vi "TelemetryServer_ChannelList.vi"(2 "error out":errorcluster, 3 "serverName":string) -> (0 "error in (no error)":errorcluster, 1 "Channel List":string[](array[string]))   [LabVIEW 2009]
uses:
  lib/lvrtc.dll
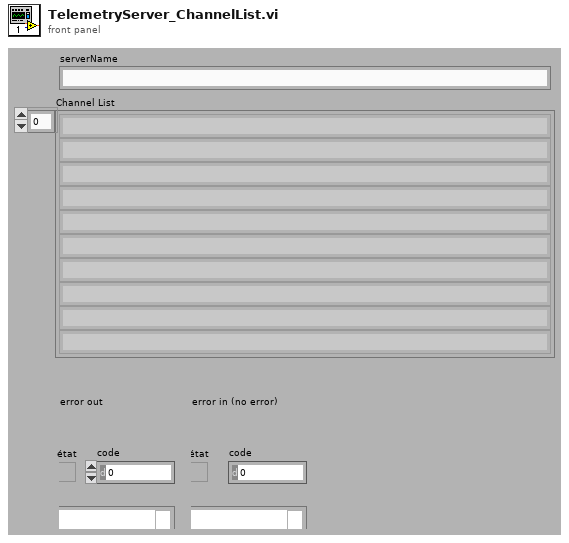
[diagram p1: front panel]
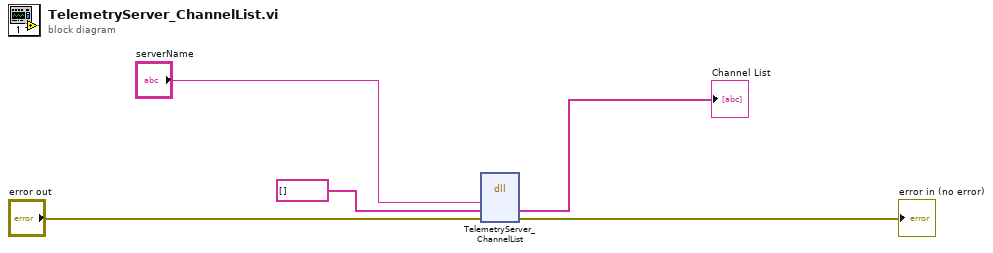
[diagram p0: block diagram]
diagram:
  n1 = dll-call lib="C:/Ohana/LV2009/OhanaOS-LV81/Instruments/RTC/Api/lib/LVRTC.dll" fn="TelemetryServer_ChannelList"("serverName"="serverName", "Channel List"=string[] [], "error out"="error out") -> ("Channel List"=→"Channel List":string[], "error out"=→"error in (no error)":errorcluster)  [unwired: 4 in, 3 out]
